vi "Vision Processing.vi"(4 "error in (no error)":errorcluster) -> ()   [LabVIEW 2013]
doc: "This VI runs in parallel to other tasks. It gets images from the camera, processes them for color or shape and use that information to affect robot behavior."
uses:
  <vilib>/Rock Robotics/WPI/Camera/WPI_CameraWhite Balance Values.ctl
  <vilib>/Rock Robotics/WPI/Camera/WPI_CameraExposure Values.ctl
  <vilib>/Rock Robotics/WPI/Camera/WPI_CameraFrameRate.ctl
  Robot Global Data.vi
panel:
  out "error out":errorcluster
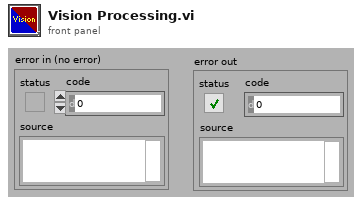
[diagram p1: front panel]
types:
  T1 = typedef "WPI_CameraFrameRate.ctl" = u32
  T2 = typedef "WPI_CameraExposure Values.ctl" = enum16{"Auto", "Flicker-free 50 Hz", "Flicker-free 60 Hz", "Hold current"}
  T3 = typedef "WPI_CameraWhite Balance Values.ctl" = enum16{"Auto", "Fixed indoor", "Fixed outdoor 1", "Fixed outdoor 2", "Fixed fluorescent 1", "Fixed fluorescent 2", "Hold current"}
  T4 = typedef "Image Type" = u32
  T5 = typedef "WPI_CameraImageSize.ctl" = enum16{"640x480", "320x240", "160x120"}
  T6 = typedef "WPI_CameraDevRef.ctl" = cluster{"Camera Address":string, "CameraStatus":errorcluster, "Acquire Image Notifier":refnum<notifier>}
  T7 = typedef "IMAQ Image.ctl" = refnum<image>
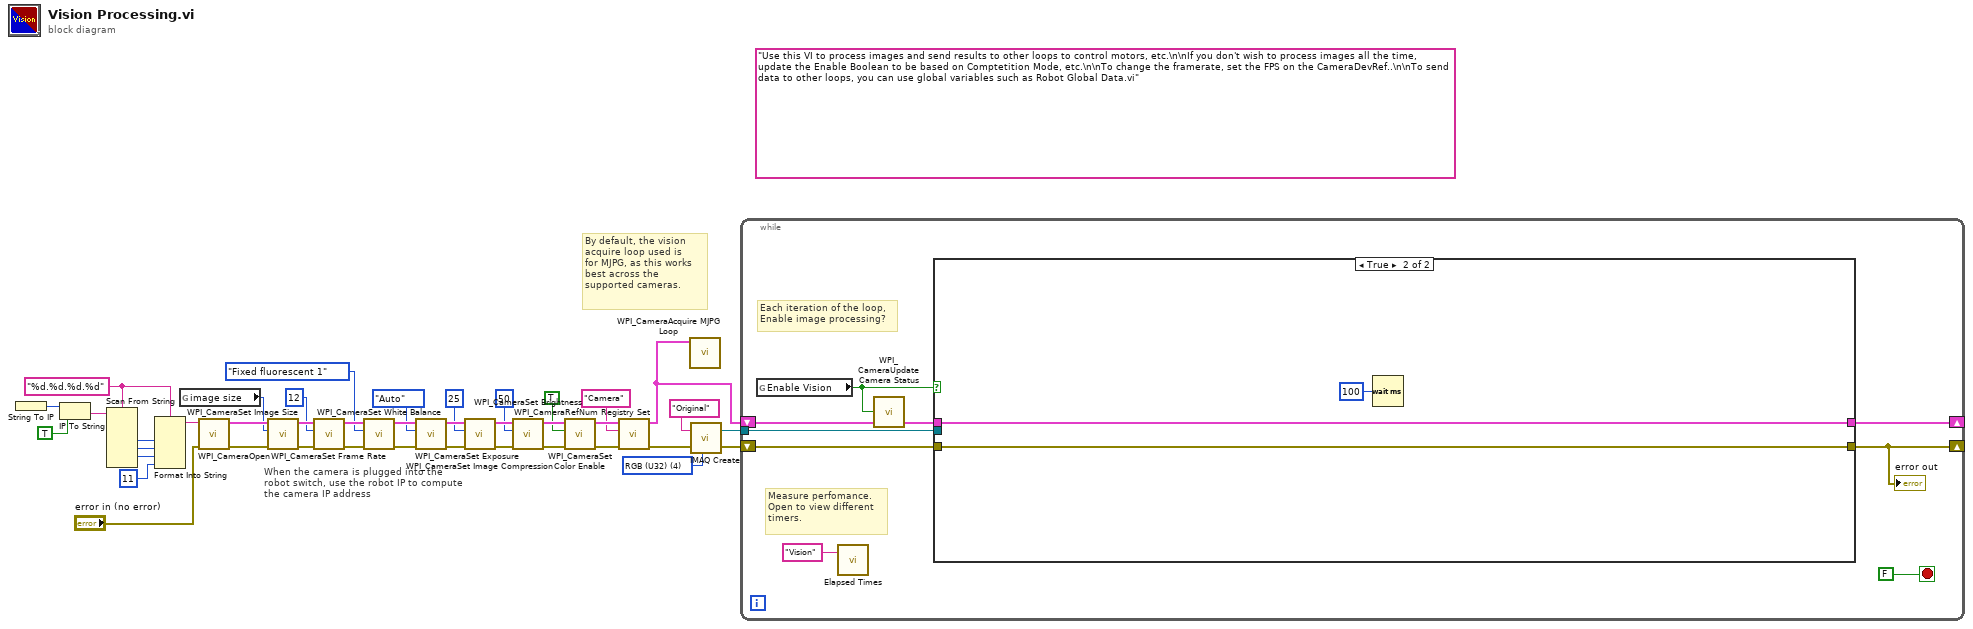
[diagram p0: block diagram]
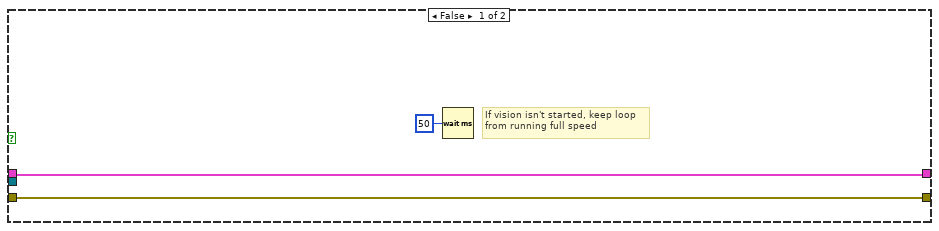
[diagram p2: hidden frame]
diagram:
  w20 = "%d.%d.%d.%d" ("format string")
  (unwired) "Use this VI to process images and send results to other loops to control motors, etc.\n\nIf you don't wish to process images all the time, update the Enable Boolean to be based on Comptetition Mode, etc.\n\nTo change the framerate, set the FPS on the CameraDevRef..\n\nTo send data to other loops, you can use global variables such as Robot Global Data.vi"
  w14 = T4 4 items=["Grayscale (U8)", "Grayscale (I16)", "Grayscale (SGL)", "Complex (CSG)", "RGB (U32)", "HSL (U32)", "RGB (U64)"] ("Image Type")
  # "When the camera is plugged into the\nrobot switch, use the robot IP to compute\nthe camera IP address"
  # "By default, the vision\nacquire loop used is\nfor MJPG, as this works\nbest across the\nsupported cameras."
  n1 = String To IP() -> (0:w27:u32)  [unwired: 1 in]
  n2 = IP To String(1:TRUE ("dot notation? (F)"), 2:w27) -> (0:w25:string)
  n3 = Scan From String(format string=w20, input string=w25) -> (output 1=w24:i32, output 2=w23:i32, output 3=w22:i32)  [unwired: 7 in, 3 out]
  n4 = Format Into String(format string=w20, w24, w23, w22, 11 ("Compression")) -> (resulting string=w19:string)  [unwired: 2 in, 1 out]
  n5 = global read "Robot Global Data.vi" "image size"() -> (w1:T5)
  n6 = call <vilib>:"WPI_CameraOpen.vi"("error in (no error)"="error in (no error)", "Camera Address"=w19) -> ("error out"=w8:errorcluster, "CameraDevRef"=w9:T6)  [unwired: 8 out]
  n7 = call <vilib>:"WPI_CameraSet Image Size.vi"("error in (no error)"=w8, "Image Size"=w1, "CameraDevRef"=w9) -> ("error out"=w35:errorcluster, "CameraDevRef Out"=w36:T6)  [unwired: 7 out]
  n8 = call <vilib>:"WPI_CameraSet Frame Rate.vi"("error in (no error)"=w35, "Frame Rate (fps)"=T1 12, "CameraDevRef"=w36) -> ("error out"=w34:errorcluster, "CameraDevRef Out"=w38:T6)  [unwired: 7 out]
  n9 = call <vilib>:"WPI_CameraSet White Balance.vi"("error in (no error)"=w34, "White Balance"=WPI_CameraWhite_Balance_Values."Fixed fluorescent 1", "CameraDevRef"=w38) -> ("error out"=w33:errorcluster, "CameraDevRef Out"=w37:T6)  [unwired: 7 out]
  n10 = call <vilib>:"WPI_CameraSet Exposure.vi"("error in (no error)"=w33, "Exposure"=WPI_CameraExposure_Values."Auto", "CameraDevRef"=w37) -> ("error out"=w32:errorcluster, "CameraDevRef Out"=w40:T6)  [unwired: 7 out]
  n11 = call <vilib>:"WPI_CameraSet Image Compression.vi"("error in (no error)"=w32, "Compression"=25, "CameraDevRef"=w40) -> ("error out"=w31:errorcluster, "CameraDevRef Out"=w39:T6)  [unwired: 7 out]
  n12 = call <vilib>:"WPI_CameraSet Brightness.vi"("error in (no error)"=w31, "Brightness"=50, "CameraDevRef"=w39) -> ("error out"=w6:errorcluster, "CameraDevRef Out"=w7:T6)  [unwired: 7 out]
  n13 = call <vilib>:"WPI_CameraSet Color Enable.vi"("error in (no error)"=w6, "Color Enabled"=TRUE, "CameraDevRef"=w7) -> ("error out"=w4:errorcluster, "CameraDevRef Out"=w5:T6)  [unwired: 7 in]
  n14 = call <vilib>:"WPI_CameraRefNum Registry Set.vi"("error in (no error)"=w4, "refnum name"="Camera", "CameraDevRef"=w5) -> ("error out"=w13:errorcluster, "CameraDevRef"=w10:T6)  [unwired: 7 out]
  n15 = call <vilib>:"WPI_CameraAcquire MJPG Loop.vi"("CameraDevRef"=w10) -> ()  [unwired: 11 in]
  n16 = call "IMAQ Create"("Image Name"="Original", "Image Type"=w14, "error in (no error)"=w13) -> ("New Image"=w11:T7, "error out"=w12:errorcluster)  [unwired: 1 in, 1 out]
  n17 = while {
    shift-right: [w45] -> _
    shift-left: w10 -> [w44]
    shift-right: [w41] -> _
    shift-left: w12 -> [w43]
    tunnel: w11 -> [w42]
    stop <- FALSE stop-if-true
    # "Measure perfomance.\nOpen to view different\ntimers."
    # "Each iteration of the loop,\nEnable image processing?"
    n18 = global read "Robot Global Data.vi" "Enable Vision"() -> (w47:bool)
    n19 = call "Elapsed Times.vi"("Call Name"="Vision") -> ()  [unwired: 2 in, 1 out]
    n20 = call <vilib>:"WPI_CameraUpdate Camera Status.vi"("CameraDevRef In"=w44, "Enable Vision"=w47) -> ("CameraDevRef Out"=w48:T6)  [unwired: 3 in]
    n21 = case shown="True" w47 {
      tunnel: w48 -> [w51 w55]
      tunnel: [w51 w55] -> w45
      tunnel: w43 -> [w50 w54]
      tunnel: [w50 w54] -> w41
      tunnel: w42 -> [_ _]
      frame False {
        # "If vision isn't started, keep loop\nfrom running full speed"
        n22 = Wait (ms)(milliseconds to wait=u32 50) -> ()  [unwired: 1 out]
      }
      frame True {
        n23 = Wait (ms)(milliseconds to wait=u32 100) -> ()  [unwired: 1 out]
      }
    }
    "error out" <- w41
  }
